vi "velocity_reversal.vi"(6 "right":dbl, 7 "left":dbl, 8 "right":bool, 9 "left":bool, 10 "down":bool, 11 "up":bool) -> (0 "right new":dbl, 3 "left new":dbl)   [LabVIEW 2011]
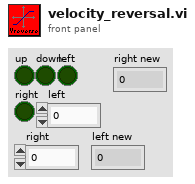
[diagram p1: front panel]
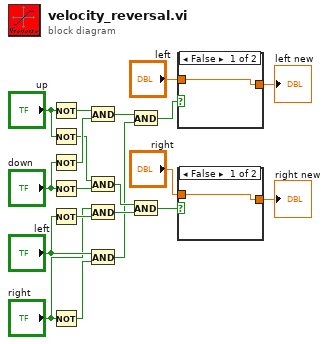
[diagram p0: block diagram]
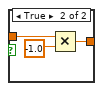
[diagram p2: hidden frame]
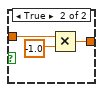
[diagram p3: hidden frame]
diagram:
  n1 = Not(x="up") -> (.not. x?=w20:bool)
  n2 = Not(x="up") -> (.not. x?=w17:bool)
  n3 = Not(x="down") -> (.not. x?=w19:bool)
  n4 = Not(x="down") -> (.not. x?=w16:bool)
  n5 = Not(x="left") -> (.not. x?=w15:bool)
  n6 = Not(x="right") -> (.not. x?=w18:bool)
  n7 = And(x=w20, y=w19) -> (x .and. y?=w12:bool)
  n8 = And(x=w17, y=w16) -> (x .and. y?=w14:bool)
  n9 = And(x="right", y=w15) -> (x .and. y?=w13:bool)
  n10 = And(x="left", y=w18) -> (x .and. y?=w11:bool)
  n11 = And(x=w12, y=w11) -> (x .and. y?=w10:bool)
  n12 = And(x=w14, y=w13) -> (x .and. y?=w9:bool)
  n13 = case shown="False" w10 {
    tunnel: "left" -> [w21 w24]
    tunnel: [w21 w22] -> w1
    frame False {
    }
    frame True {
      n14 = Multiply(x=w24, y=-1.0) -> (x*y=w22:dbl)
    }
  }
  "left new" <- w1
  n15 = case shown="False" w9 {
    tunnel: [w25 w27] -> w3
    tunnel: "right" -> [w25 w26]
    frame False {
    }
    frame True {
      n16 = Multiply(x=w26, y=-1.0) -> (x*y=w27:dbl)
    }
  }
  "right new" <- w3
